vi "Ejercicios Array.vi"() -> ()   [LabVIEW 2010]
panel:
  out "x+y 3":dbl[](array[numeric])
  out "x+y 2":dbl[](array[numeric])
  out "x+y":dbl[](array[numeric])
  out "subarray 2":dbl[](array[numeric])
  out "element":dbl
  out "appended array 3":dbl[](array[numeric])
  out "appended array 2":dbl[][](array[numeric])
  out "appended array":dbl[](array[numeric])
  out "subarray":dbl[](array[numeric])
  out "initialized array":dbl[](array[numeric])
  out "size":i32
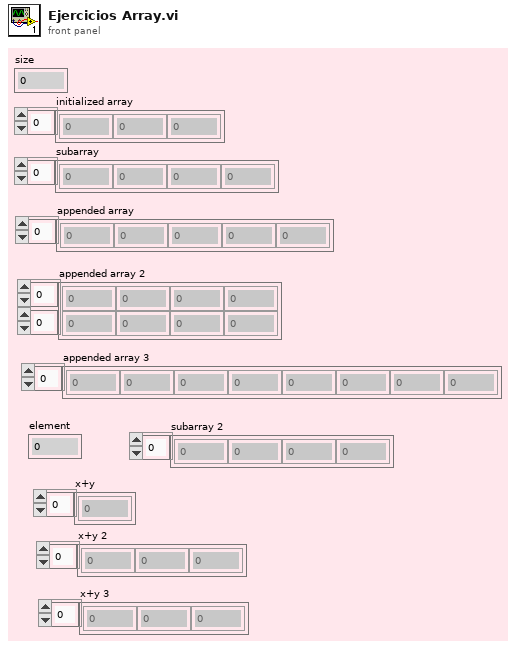
[diagram p1: front panel]
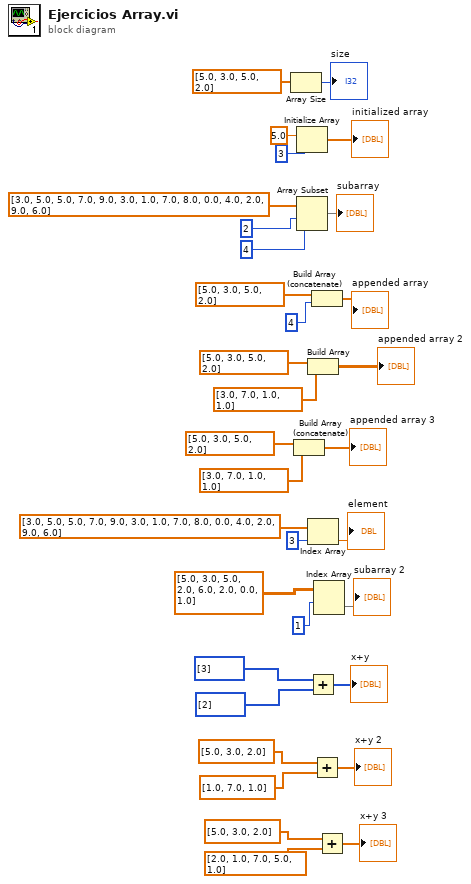
[diagram p0: block diagram]
diagram:
  n1 = Array Size(array=dbl[] [5.0, 3.0, 5.0, 2.0]) -> (size(s)=→"size":i32)
  n2 = Build Array (concatenate)(dbl[] [5.0, 3.0, 5.0, 2.0] ("array"), dbl[] [3.0, 7.0, 1.0, 1.0] ("element")) -> (→"appended array 3":dbl[])
  n3 = Initialize Array(5.0 ("element"), 3 ("dimension size")) -> (→"initialized array":dbl[])
  n4 = Array Subset(array=dbl[] [3.0, 5.0, 5.0, 7.0, 9.0, 3.0, 1.0, 7.0, 8.0, 0.0, 4.0, 2.0, 9.0, 6.0], index=2, length=4) -> (→"subarray":dbl[])
  n5 = Build Array(dbl[] [5.0, 3.0, 5.0, 2.0] ("array"), dbl[] [3.0, 7.0, 1.0, 1.0] ("element")) -> (→"appended array 2":dbl[][])
  n6 = Index Array(array=dbl[] [3.0, 5.0, 5.0, 7.0, 9.0, 3.0, 1.0, 7.0, 8.0, 0.0, 4.0, 2.0, 9.0, 6.0], index=3) -> (element=→"element":dbl)
  n7 = Add(x=i32[] [3] ("array"), y=i32[] [2] ("element")) -> (x+y=→"x+y":i32[])
  n8 = Build Array (concatenate)(dbl[] [5.0, 3.0, 5.0, 2.0] ("array"), 4 ("length")) -> (→"appended array":dbl[])
  n9 = Add(x=dbl[] [5.0, 3.0, 2.0] ("array"), y=dbl[] [1.0, 7.0, 1.0] ("element")) -> (x+y=→"x+y 2":dbl[])
  n10 = Index Array(array=dbl[][] [[5.0, 3.0, 5.0, 2.0], [6.0, 2.0, 0.0, 1.0]], index (row)=1) -> (element=→"subarray 2":dbl[])  [unwired: 1 in]
  n11 = Add(x=dbl[] [5.0, 3.0, 2.0] ("array"), y=dbl[] [2.0, 1.0, 7.0, 5.0, 1.0] ("element")) -> (x+y=→"x+y 3":dbl[])
